vi "Init Game Pad.vi"(8 "error in (no error)":errorcluster, 11 "Hardware Game Pad Interface in":refnum<class "Hardware Game Pad Interface.lvclass">) -> (0 "error out":errorcluster, 3 "Hardware Game Pad Interface out":refnum<class "Hardware Game Pad Interface.lvclass">)   [LabVIEW 2017, in "Hardware Game Pad Interface.lvclass"]
uses:
  Hardware Game Pad Interface.lvclass
  Hardware Game Pad Interface.lvclass/Hardware Game Pad Interface.ctl
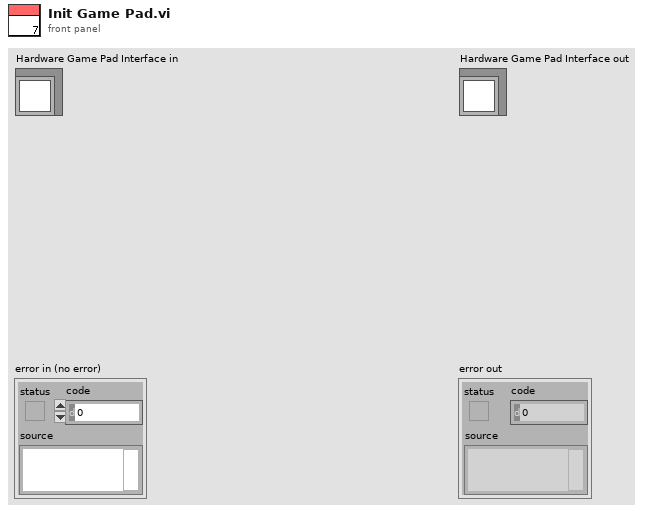
[diagram p1: front panel]
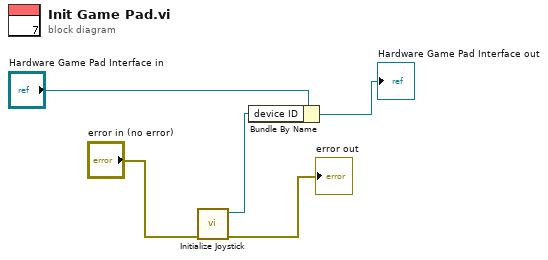
[diagram p0: block diagram]
diagram:
  n1 = call <vilib>:"Initialize Joystick.vi"("error in (no error)"="error in (no error)") -> ("error out"=→"error out":errorcluster, "device ID"=w3:refnum<k1>)  [unwired: 9 in]
  n2 = Bundle By Name(cluster="Hardware Game Pad Interface in", "device ID"=w3) -> (→"Hardware Game Pad Interface out":refnum<class "Hardware Game Pad Interface.lvclass">)
